vi "GenerateHTML.vi"(6 "Unattended Mode":bool, 8 "error in (no error)":errorcluster, 9 "Files to preload":path[](array[path]), 10 "Destination Directory":path, 11 "Source directory/files":path) -> (0 "error out":errorcluster, 3 "Output":string)   [LabVIEW 2017]
uses:
  JsonConverters/ConverterBase/FileConverterBase.lvclass
  JsonConverters/LVFileConverters/ClassConverter/ClassConverter.lvclass
  C:/FINALE/src/HTMLGenerator/JsonConverters/ConverterBase/FileConverterBase.lvclass
  JsonConverters/LVFileConverters/VIConverter/VIConverter.lvclass
  PathConfiguration.vi
panel:
  out "?":u8(slide) scale=0.0..100.0
  out "File being converted":path
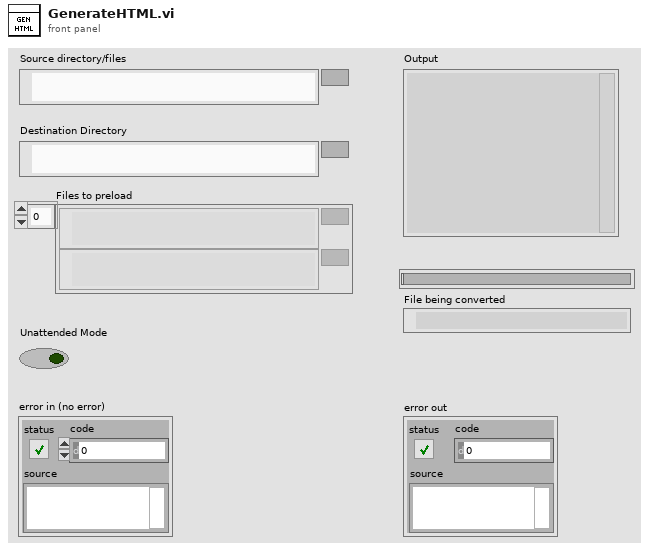
[diagram p1: front panel]
types:
  T1 = typedef "ApplicationItems.ctl" = cluster{"Application Reference":refnum<vi>, "Files":T2[]}
  T2 = typedef "SourceJsonPaths.ctl" = cluster{"File to convert":path, "Output directory":path}
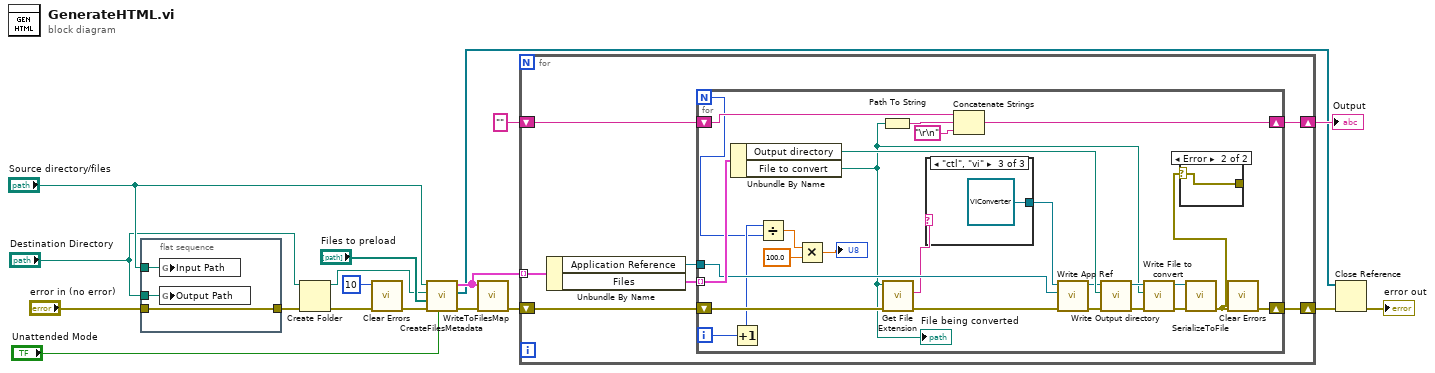
[diagram p0: block diagram]
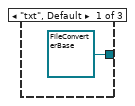
[diagram p3: hidden frame]
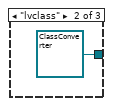
[diagram p4: hidden frame]
diagram:
  n1 = flat-sequence {
    tunnel: "Source directory/files" -> [w21]
    tunnel: "Destination Directory" -> [w20]
    tunnel: "error in (no error)" -> [w19]
    tunnel: [w19] -> w8
    frame #0 {
      n2 = global write "PathConfiguration.vi" "Input Path"(w21) -> ()
      n3 = global write "PathConfiguration.vi" "Output Path"(w20) -> ()
    }
  }
  n4 = Create Folder(path (use dialog)="Destination Directory", error in=w8) -> (created path=w9:path, error out=w7:errorcluster)  [unwired: 1 in, 1 out]
  n5 = call <vilib>:"Clear Errors.vi"("error in (no error)"=w7, "specific error code to clear (0: all)"=10) -> ("error out"=w6:errorcluster)  [unwired: 4 in, 1 out]
  n6 = call "CreateFilesMetadata.vi"("Unattended Mode"="Unattended Mode", "error in (no error)"=w6, "Files to preload"="Files to preload", "Output Directory"=w9, "Source directory/files"="Source directory/files") -> ("error out"=w14:errorcluster, "Opened file refs"=w2:refnum<vi>[], "Items To Serialize"=w12:T1[])  [unwired: 4 in]
  n7 = call "WriteToFilesMap.vi"("error in (no error)"=w14, "Items To Serialize"=w12) -> ("error out"=w13:errorcluster)  [unwired: 9 in]
  n8 = for {
    shift-right: [w27] -> w4
    shift-left: w13 -> [w28]
    tunnel: w12 -> [w26] mode=indexing
    shift-right: [w23] -> w15
    shift-left: "" -> [w24]
    n9 = Unbundle By Name(w26) -> ("Application Reference"=w25:refnum<vi>, "Files"=w22:T2[])
    n10 = for {
      N -> [w30]
      tunnel: w25 -> [w45]
      tunnel: w22 -> [w46] mode=indexing
      shift-right: [w36] -> w27
      shift-left: w28 -> [w43]
      shift-right: [w39] -> w23
      shift-left: w24 -> [w41]
      i -> [w31]
      n11 = Unbundle By Name(w46) -> ("Output directory"=w54:path, "File to convert"=w40:path)
      "File being converted" <- w40
      n12 = Increment(x=w31) -> (x+1=w34:i32)
      n13 = Divide(x=w34, y=w30) -> (x/y=w33:dbl)
      n14 = Multiply(x=w33, y=100.0) -> (x*y=→"?":dbl)
      n15 = Path To String(path=w40) -> (string=w38:string)
      n16 = call <vilib>:"Get File Extension.vi"("error in (no error)"=w43, "file"=w40) -> ("error out"=w42:errorcluster, "lowercase file extension"=w44:string)  [unwired: 5 in, 3 out]
      n17 = case shown="\"ctl\", \"vi\"" w44 {
        tunnel: [refnum<class "FileConverterBase.lvclass"> refnum ("FileConverterBase.lvclass") refnum<class "ClassConverter.lvclass"> refnum ("ClassConverter.lvclass") refnum<class "VIConverter.lvclass"> refnum ("VIConverter.lvclass")] -> w53
        frame "txt", Default {
        }
        frame "lvclass" {
        }
        frame "ctl", "vi" {
        }
      }
      n18 = Concatenate Strings(w41, w38, "\r\n") -> (w39:string)
      n19 = call-dynamic "Write App Ref.vi"("error in (no error)"=w42, "App Ref"=w45, "FileConverterBase in"=w53) -> ("error out"=w47:errorcluster, "FileConverterBase out"=w52:refnum<class "FileConverterBase.lvclass">)  [unwired: 7 in]
      n20 = call-dynamic "Write Output directory.vi"("error in (no error)"=w47, "Output JSON File Path"=w54, "FileConverterBase in"=w52) -> ("error out"=w48:errorcluster, "FileConverterBase out"=w51:refnum<class "FileConverterBase.lvclass">)  [unwired: 7 in]
      n21 = call-dynamic "Write File to convert.vi"("error in (no error)"=w48, "Input File Path"=w40, "FileConverterBase in"=w51) -> ("error out"=w49:errorcluster, "FileConverterBase out"=w50:refnum<class "FileConverterBase.lvclass">)  [unwired: 7 in]
      n22 = call-dynamic "SerializeToFile.vi"("error in (no error)"=w49, "FileConverterBase in"=w50) -> ("error out"=w35:errorcluster)  [unwired: 8 in, 1 out]
      n23 = case shown="Error" w35 {
        selector: w35 -> [w55 w56]
        tunnel: [w55 w56] -> _
        frame No Error {
        }
        frame Error {
        }
      }
      n24 = call <vilib>:"Clear Errors.vi"("error in (no error)"=w35) -> ("error out"=w36:errorcluster)  [unwired: 5 in, 1 out]
    }
  }
  "Output" <- w15
  n25 = Close Reference(reference=w2, error in (no error)=w4) -> (error out=→"error out":errorcluster)
